vi "loadOvenDataToOvenLot.vi"() -> ()   [LabVIEW 2012]
uses:
  <vilib>/addons/database/Connection.llb/DB Tools Open Connec (Path).vi
  <vilib>/addons/database/Connection.llb/Conn Execute.vi
  <vilib>/addons/database/Recordset.llb/Rec Fetch Recordset Data (R).vi
  <vilib>/addons/database/Recordset.llb/Rec Destroy - Connection.vi
  <vilib>/addons/database/_DB Variant To Data/Database Variant To Data.xnode
  <vilib>/addons/database/NI_Database_API.lvlib
panel:
  out "data":string
  in  "input cluster":cluster{"rc":string, "lots":string}
  out "error out":errorcluster
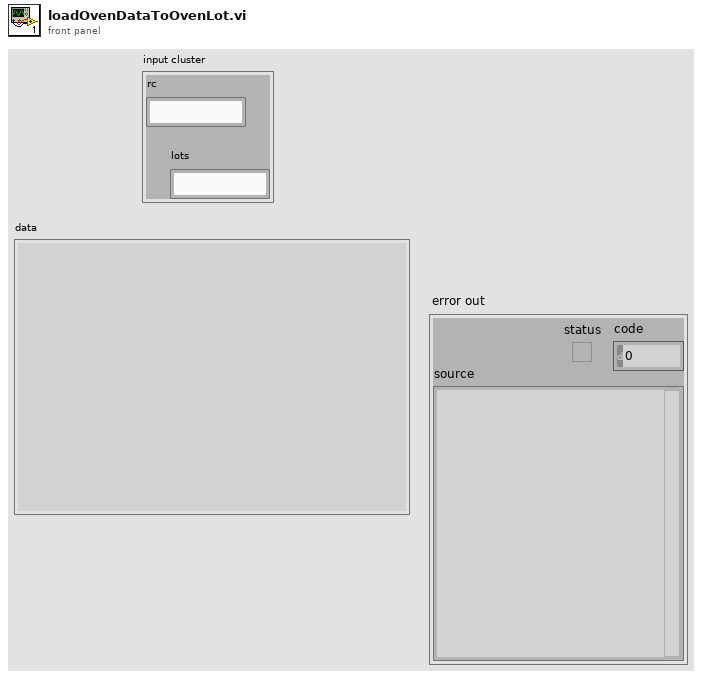
[diagram p1: front panel]
types:
  T1 = typedef "NI_Database_API.lvlib/Conn ObjectReference.ctl" = refnum<k1>
  T2 = typedef "NI_Database_API.lvlib/Rec ObjectReference.ctl" = refnum<k1>
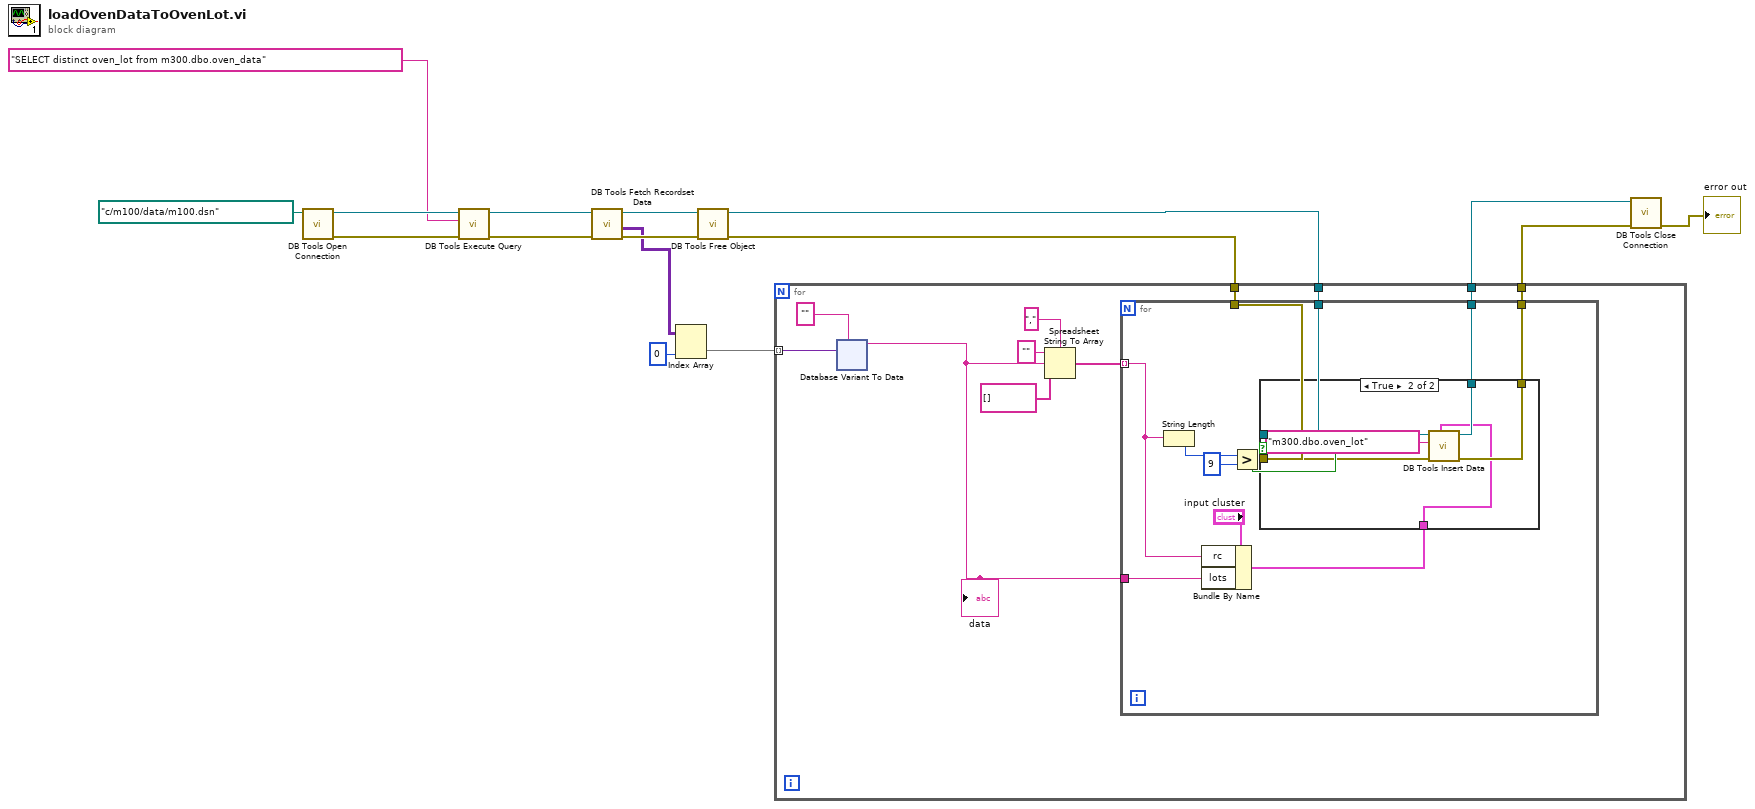
[diagram p0: block diagram]
diagram:
  n1 = call-poly <vilib>:"DB Tools Open Connection.vi"("connection information"=path "c:/m100/data/m100.dsn") -> ("error out"=w15:errorcluster, "connection reference"=w16:T1)  [unwired: 7 in]
  n2 = call-poly <vilib>:"DB Tools Execute Query.vi"("error in (no error)"=w15, "SQL query"="SELECT distinct oven_lot from m300.dbo.oven_data", "connection reference"=w16) -> ("error out"=w13:errorcluster, "recordset reference"=w14:T2)  [unwired: 5 in]
  n3 = call-poly <vilib>:"DB Tools Fetch Recordset Data.vi"("error in (no error)"=w13, "recordset reference"=w14) -> ("error out"=w11:errorcluster, "recordset data"=w7:variant[][], "recordset reference out"=w12:T2)  [unwired: 3 in]
  n4 = Index Array(array=w7, index (col)=0 ("disabled index (col)")) -> (element=w5:variant[])  [unwired: 1 in]
  n5 = call-poly <vilib>:"DB Tools Free Object.vi"("error in (no error)"=w11, "recordset reference"=w12) -> ("error out"=w3:errorcluster, "connection reference"=w4:T1)  [unwired: 8 in]
  n6 = for {
    tunnel: w5 -> [w24] mode=indexing
    tunnel: w4 -> [w21]
    tunnel: w3 -> [w20]
    tunnel: [w19] -> w2
    tunnel: [w18] -> w1
    n7 = xnode "Database Variant To Data"("database variant"=w24, "type"="") -> ("data"=w17:string)  [unwired: 1 in, 1 out]
    "data" <- w17
    n8 = Spreadsheet String To Array(delimiter (Tab)=",", format string="", spreadsheet string=w17, array type (2D Dbl)=string[] []) -> (array=w22:string[])
    n9 = for {
      tunnel: w22 -> [w30] mode=indexing
      tunnel: w21 -> [w36]
      tunnel: w20 -> [w35]
      tunnel: [w34] -> w19
      tunnel: [w33] -> w18
      tunnel: w17 -> [w29]
      n10 = String Length(string=w30) -> (length=w38:i32)
      n11 = Bundle By Name(cluster="input cluster", "rc"=w30, "lots"=w29) -> (w28:cluster{"rc":string, "lots":string})
      n12 = Greater?(x=w38, y=9) -> (0:w32:bool)
      n13 = case shown="True" w32 {
        tunnel: w36 -> [w40 w46]
        tunnel: w35 -> [w39 w45]
        tunnel: [w40 w44] -> w34
        tunnel: [w39 w43] -> w33
        tunnel: w28 -> [_ w41]
        frame False {
        }
        frame True {
          n14 = call <vilib>:"DB Tools Insert Data.vi"("data"=w41, "error in (no error)"=w45, "table"="m300.dbo.oven_lot", "connection reference"=w46) -> ("error out"=w43:errorcluster, "connection reference out"=w44:T1)  [unwired: 6 in]
        }
      }
    }
  }
  n15 = call <vilib>:"DB Tools Close Connection.vi"("error in (no error)"=w1, "connection reference"=w2) -> ("error out"=→"error out":errorcluster)  [unwired: 5 in]
